vi "Hanging.vi"(9 "Pneumatics In":T2={"CompressorDevRef"={"DevStatus"={"status"=FALSE, "code"=0, "source"=""}, "Pneumatics Control Module"=0}, "High and Low Gear DoubleSolenoidDevRef"={"DevStatus"={"status"=FALSE, "code"=0, "source"=""}, "Pneumatics Control Module"=0, "Forward Solenoid Channel"=enum."Invalid", "Reverse Solenoid Channel"=enum."Invalid"}, "PTO SolenoidDevRef"={"DevStatus"={"status"=FALSE, "code"=0, "source"=""}, "Pneumatics Control Module"=0, "Forward Solenoid Channel"=enum."Invalid", "Reverse Solenoid Channel"=enum."Invalid"}, "Hang Pin SolenoidDevRef"={"DevStatus"={"status"=FALSE, "code"=0, "source"=""}, "Pneumatics Control Module"=0, "Forward Solenoid Channel"=enum."Invalid", "Reverse Solenoid Channel"=enum."Invalid"}}, 11 "Hanging":T13={"Left Erection MotorControlDeviceRef"={"DeviceStatus"={"status"=FALSE, "code"=0, "source"=""}, "Type"=enum."PWM", "PWM"={"PWM Channel"=enum."Invalid", "DeadBand"={"Name"="", "maxPositivePwm"=0, "minPositivePwm"=0, "centerPwm"=0, "maxNegativePwm"=0, "minNegativePwm"=0, "angularRange"=0}}, "CAN"={"Device Number"=0, "Control Mode"=enum."Percent VBus", "Semaphore"=refnum, "Max Vout"=12.0, "TalonSRX Control Mode"=enum."Percent VBus"}, "Invert"=FALSE}, "Right Erection MotorControlDeviceRef"={"DeviceStatus"={"status"=FALSE, "code"=0, "source"=""}, "Type"=enum."PWM", "PWM"={"PWM Channel"=enum."Invalid", "DeadBand"={"Name"="", "maxPositivePwm"=0, "minPositivePwm"=0, "centerPwm"=0, "maxNegativePwm"=0, "minNegativePwm"=0, "angularRange"=0}}, "CAN"={"Device Number"=0, "Control Mode"=enum."Percent VBus", "Semaphore"=refnum, "Max Vout"=12.0, "TalonSRX Control Mode"=enum."Percent VBus"}, "Invert"=FALSE}}) -> (1 "Pneumatics Out":T2={"CompressorDevRef"={"DevStatus"={"status"=FALSE, "code"=0, "source"=""}, "Pneumatics Control Module"=0}, "High and Low Gear DoubleSolenoidDevRef"={"DevStatus"={"status"=FALSE, "code"=0, "source"=""}, "Pneumatics Control Module"=0, "Forward Solenoid Channel"=enum."Invalid", "Reverse Solenoid Channel"=enum."Invalid"}, "PTO SolenoidDevRef"={"DevStatus"={"status"=FALSE, "code"=0, "source"=""}, "Pneumatics Control Module"=0, "Forward Solenoid Channel"=enum."Invalid", "Reverse Solenoid Channel"=enum."Invalid"}, "Hang Pin SolenoidDevRef"={"DevStatus"={"status"=FALSE, "code"=0, "source"=""}, "Pneumatics Control Module"=0, "Forward Solenoid Channel"=enum."Invalid", "Reverse Solenoid Channel"=enum."Invalid"}}, 3 "Hanging":T13={"Left Erection MotorControlDeviceRef"={"DeviceStatus"={"status"=FALSE, "code"=0, "source"=""}, "Type"=enum."PWM", "PWM"={"PWM Channel"=enum."Invalid", "DeadBand"={"Name"="", "maxPositivePwm"=0, "minPositivePwm"=0, "centerPwm"=0, "maxNegativePwm"=0, "minNegativePwm"=0, "angularRange"=0}}, "CAN"={"Device Number"=0, "Control Mode"=enum."Percent VBus", "Semaphore"=refnum, "Max Vout"=12.0, "TalonSRX Control Mode"=enum."Percent VBus"}, "Invert"=FALSE}, "Right Erection MotorControlDeviceRef"={"DeviceStatus"={"status"=FALSE, "code"=0, "source"=""}, "Type"=enum."PWM", "PWM"={"PWM Channel"=enum."Invalid", "DeadBand"={"Name"="", "maxPositivePwm"=0, "minPositivePwm"=0, "centerPwm"=0, "maxNegativePwm"=0, "minNegativePwm"=0, "angularRange"=0}}, "CAN"={"Device Number"=0, "Control Mode"=enum."Percent VBus", "Semaphore"=refnum, "Max Vout"=12.0, "TalonSRX Control Mode"=enum."Percent VBus"}, "Invert"=FALSE}})   [LabVIEW 2015]
uses:
  <vilib>/Rock Robotics/WPI/MotorControl/WPI_MotorControlDeviceRef.ctl
  <vilib>/Rock Robotics/WPI/MotorControl/WPI_MotorControlType.ctl
  <vilib>/Rock Robotics/SystemInterfaces/DIO/FPGA_DIOPWMChannel.ctl
  <vilib>/Rock Robotics/WPI/PWM/WPI_PWMDeadband.ctl
  <vilib>/Rock Robotics/WPI/CAN/Jaguar/SubVIs/WPI_CANJaguar_ControlMode.ctl
  <vilib>/Rock Robotics/WPI/CAN/TalonSRX/WPI_CANTalonSRX_APIControlMode.ctl
  Pnematics.ctl
  <vilib>/Rock Robotics/WPI/Compressor/WPI_CompressorDevRef.ctl
  <vilib>/Rock Robotics/WPI/Solenoid/WPI_SolenoidDevRef.ctl
  <vilib>/Rock Robotics/WPI/Solenoid/WPI_SolenoidChannel.ctl
  <vilib>/Rock Robotics/WPI/Solenoid/WPI_SolenoidValue.ctl
  Robot Values.vi
  <vilib>/Rock Robotics/Network Tables/NT Write String.vi
  <vilib>/Rock Robotics/WPI/Solenoid/WPI_SolenoidSetEnum.vi
  <vilib>/ptbypt/NI_PtbyPt.lvlib
panel:
  out "Right pivot encoder":dbl
  out "Left pivot encoder":dbl
  in  "Pin In":T1=enum."Reverse"
  in  "Pin Out":T1=enum."Forward"
  in  "PTO OUT":T1=enum."Forward"
  in  "PTO IN":T1=enum."Reverse"
  out "encoder offset":dbl
  in  "Setpoint":dbl=100.0
  # "THESE VALUES NEED TO BE UPDATED"
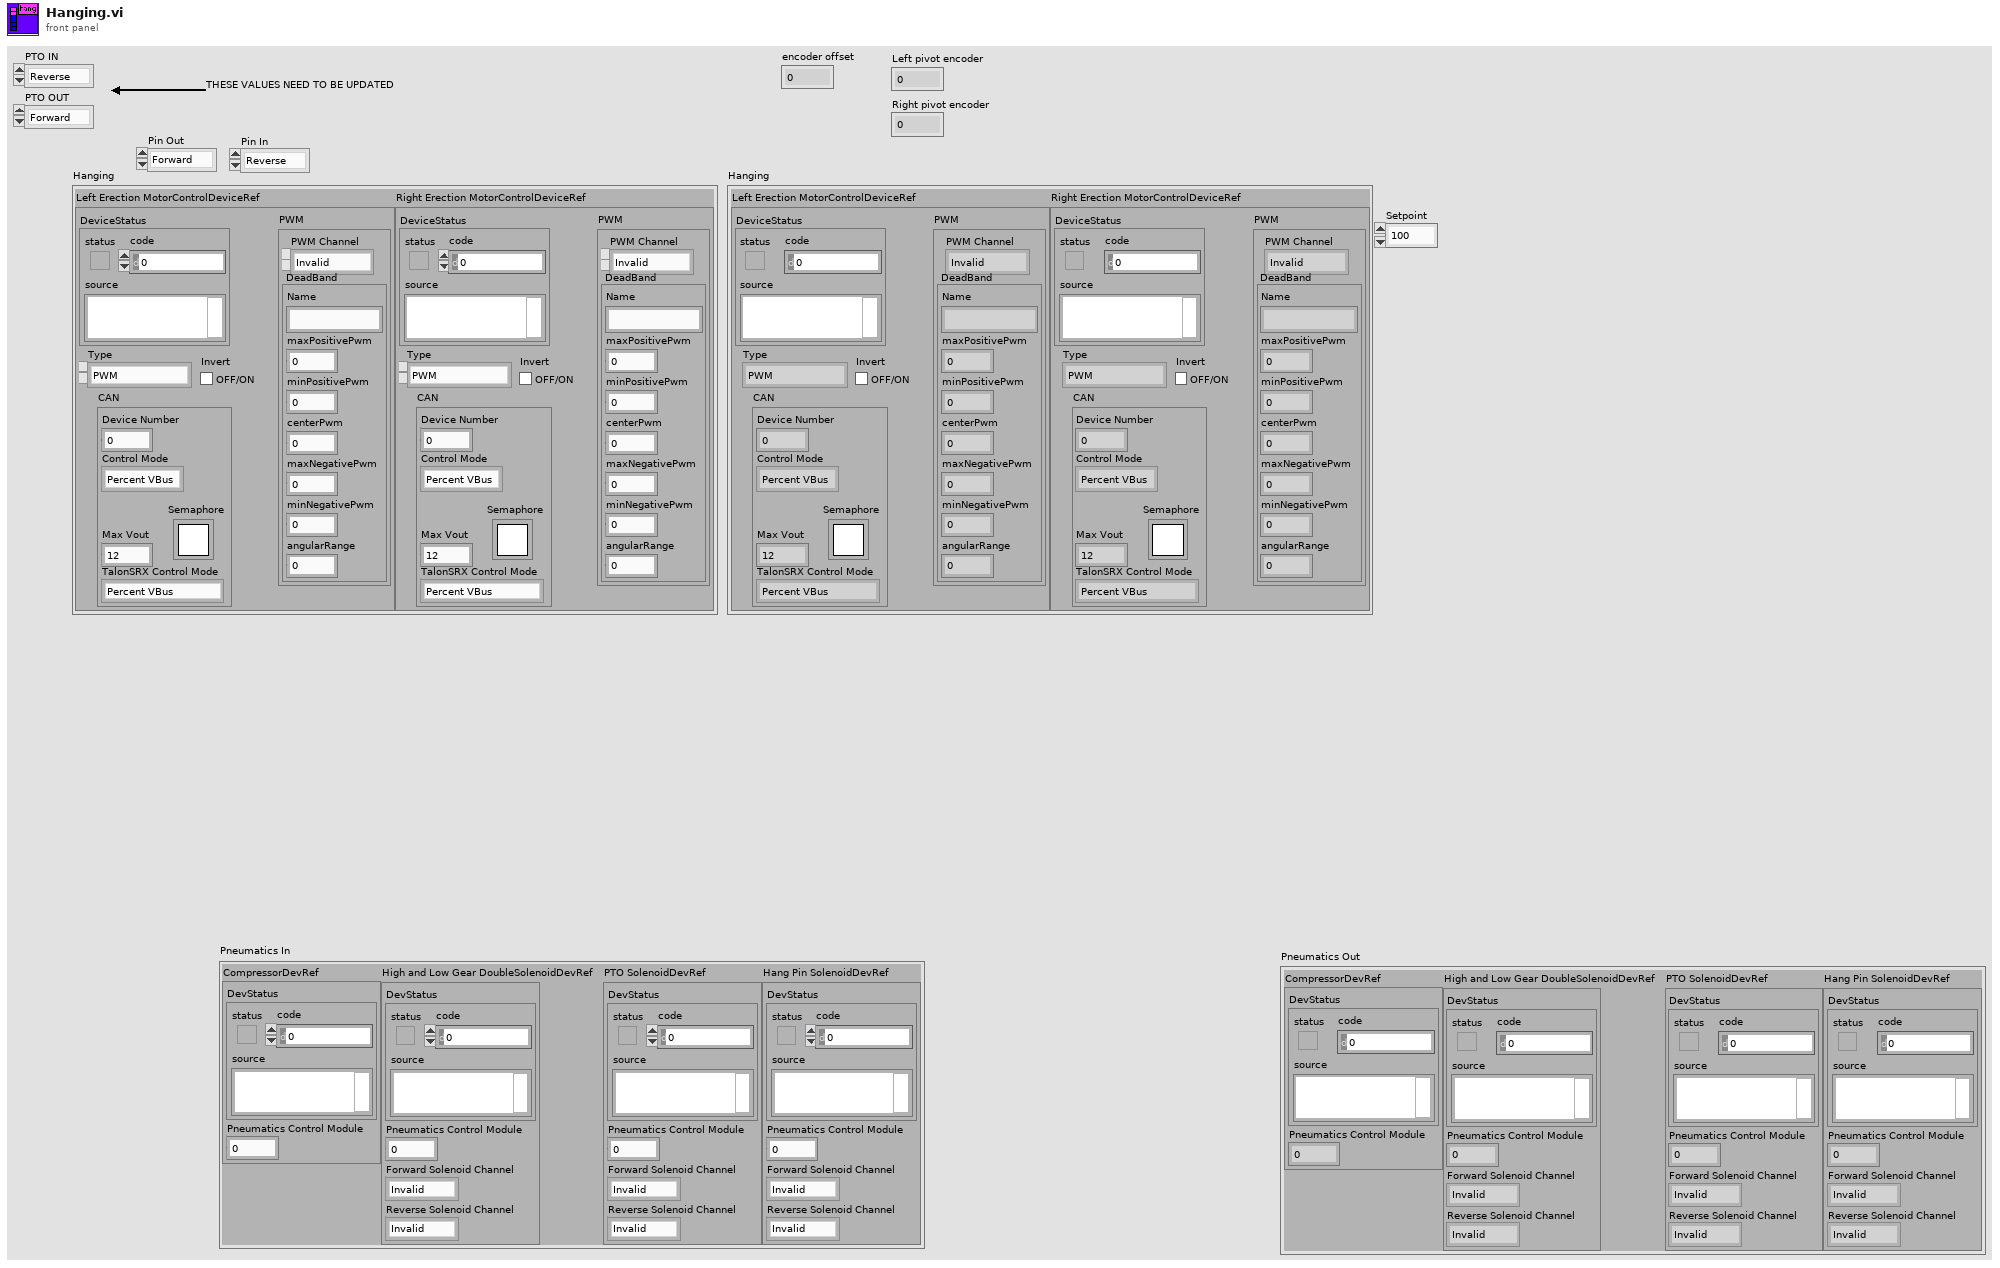
[diagram p1: front panel]
types:
  T1 = typedef "WPI_SolenoidValue.ctl" = enum16{"Off", "On", "Forward", "Reverse"}
  T2 = typedef "Pnematics.ctl" = cluster{"CompressorDevRef":T3, "High and Low Gear DoubleSolenoidDevRef":T4, "PTO SolenoidDevRef":T4, "Hang Pin SolenoidDevRef":T4}
  T3 = typedef "WPI_CompressorDevRef.ctl" = cluster{"DevStatus":errorcluster, "Pneumatics Control Module":u8}
  T4 = typedef "WPI_SolenoidDevRef.ctl" = cluster{"DevStatus":errorcluster, "Pneumatics Control Module":u8, "Forward Solenoid Channel":T5, "Reverse Solenoid Channel":T5}
  T5 = typedef "WPI_SolenoidChannel.ctl" = enum8{"Solenoid 0", "Solenoid 1", "Solenoid 2", "Solenoid 3", "Solenoid 4", "Solenoid 5", "Solenoid 6", "Solenoid 7", "Invalid"}
  T6 = typedef "WPI_MotorControlDeviceRef.ctl" = cluster{"DeviceStatus":errorcluster, "Type":T7, "PWM":cluster{"PWM Channel":T8, "DeadBand":T9}, "CAN":cluster{"Device Number":u8, "Control Mode":T10, "Semaphore":T11, "Max Vout":dbl, "TalonSRX Control Mode":T12}, "Invert":bool}
  T7 = typedef "WPI_MotorControlType.ctl" = enum16{"PWM", "CAN", "CANTalonSRX"}
  T8 = typedef "FPGA_DIOPWMChannel.ctl" = enum8{"PWM 0", "PWM 1", "PWM 2", "PWM 3", "PWM 4", "PWM 5", "PWM 6", "PWM 7", "PWM 8", "PWM 9", "PWM MXP 0", "PWM MXP 1", "PWM MXP 2", "PWM MXP 3", "PWM MXP 4", "PWM MXP 5", "PWM MXP 6", "PWM MXP 7", "PWM MXP 8", "PWM MXP 9", "Invalid"}
  T9 = typedef "WPI_PWMDeadband.ctl" = cluster{"Name":string, "maxPositivePwm":i32, "minPositivePwm":i32, "centerPwm":i32, "maxNegativePwm":i32, "minNegativePwm":i32, "angularRange":u16}
  T10 = typedef "WPI_CANJaguar_ControlMode.ctl" = enum8{"Percent VBus", "Current", "Speed", "Position", "Voltage"}
  T11 = typedef "Semaphore RefNum" = refnum<k1>
  T12 = typedef "WPI_CANTalonSRX_APIControlMode.ctl" = enum8{"Percent VBus", "Speed", "Position", "Slave", "Unchanged / Invalid", "Voltage Compensation", "Current", "Motion Profile"}
  T13 = cluster{"Left Erection MotorControlDeviceRef":T6, "Right Erection MotorControlDeviceRef":T6}
  T14 = typedef "Robot Values.ctl" = cluster{"Drive Motors":cluster{"Left Motor Value":dbl, "Right Motor Value":dbl, "Left Motor Encoder":dbl, "Right Motor Encoder":dbl, "High/Low Gear":bool}, "Sensors":cluster{"Gyro Angle":dbl, "Photoeye":bool, "Ultrasonic Range":dbl, "Shooter Speed Encoder":dbl, "Accelerometer Value":dbl, "Flashlight":bool, "Target Distance":dbl, "Target X Value":dbl, "Reset Gyro?":bool}, "Arms":cluster{"Desired Arm Position":dbl, "Left Arm Encoder":dbl, "Right Arm Encoder":dbl, "Left Arm Lower Limit":bool, "Right Arm Lower Limit":bool, "Initialize Arm Position?":bool}, "Acquisition and Scoring":cluster{"Acquiring?":bool, "Current Speed":dbl, "Setpoint Speed":dbl, "Prep Wheels":bool, "Shoot":bool, "Low Eject":bool, "Reverse Shooter Wheel":bool}, "Hanging":cluster{"Pivot Arms":dbl, "PTO":bool, "Left Pivot Encoder":dbl, "Right Pivot Encoder":dbl, "Hanging Pin":bool}}
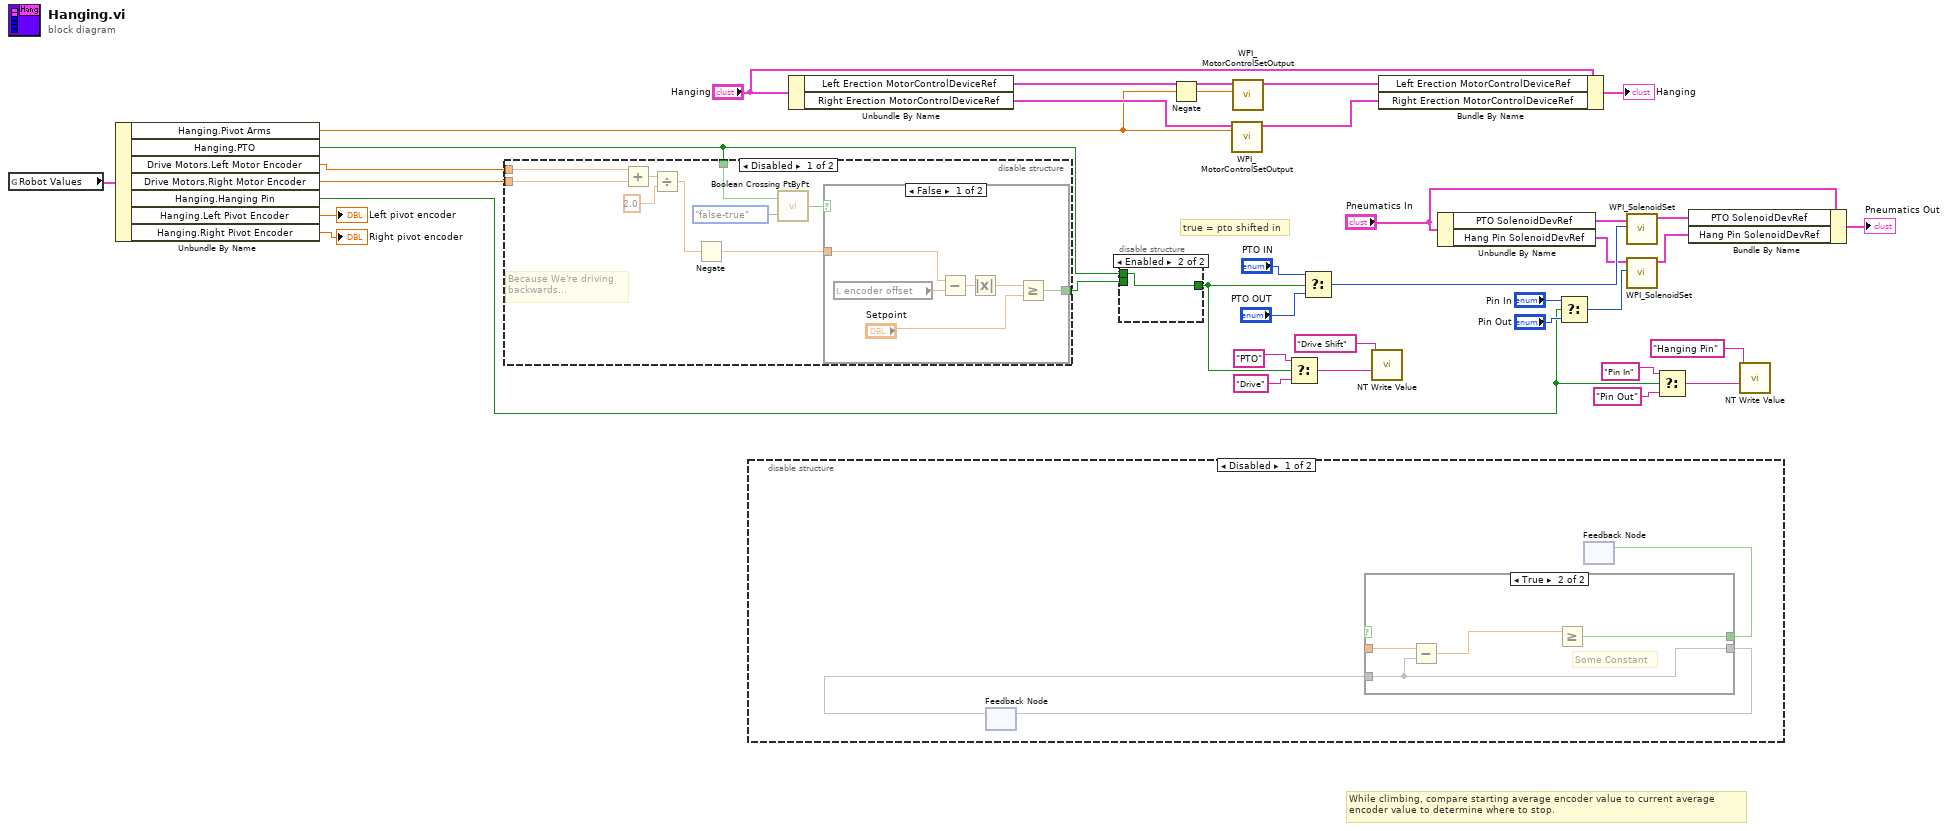
[diagram p0: block diagram]
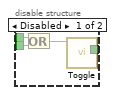
[diagram p2: hidden frame]
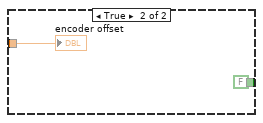
[diagram p3: hidden frame]
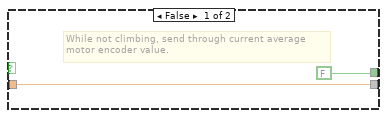
[diagram p5: hidden frame]
diagram:
  # "true = pto shifted in"
  # "While climbing, compare starting average encoder value to current average\nencoder value to determine where to stop."
  n1 = global read "Robot Values.vi" "Robot Values"() -> (w31:T14)
  n2 = Unbundle By Name(w31) -> ("Hanging.Pivot Arms"=w30:dbl, "Hanging.PTO"=w17:bool, "Drive Motors.Left Motor Encoder"=w22:dbl, "Drive Motors.Right Motor Encoder"=w21:dbl, "Hanging.Hanging Pin"=w1:bool, "Hanging.Left Pivot Encoder"=→"Left pivot encoder":dbl, "Hanging.Right Pivot Encoder"=→"Right pivot encoder":dbl)
  n3 = disable-structure shown="Disabled" {
    disable-tunnel: w22 -> [w47 _]
    disable-tunnel: w21 -> [w46 _]
    disable-tunnel: w17 -> [w43 _]
    disable-tunnel: [w40 _] -> w16
    frame Disabled {
      # "Because We're driving \nbackwards..."
      n4 = Add(x=w47, y=w46) -> (x+y=w45:dbl)
      n5 = Divide(x=w45, y=2.0) -> (x/y=w39:dbl)
      n6 = Negate(x=w39) -> (-x=w38:dbl)
      n7 = call <vilib>:"Boolean Crossing PtByPt.vi"("direction"=enum16{"either", "false-true", "true-false"}."false-true", "input"=w43) -> ("crossing"=w41:bool)  [unwired: 1 in]
      n8 = case shown="False" w41 {
        tunnel: w38 -> [w52 w55]
        tunnel: [w50 FALSE] -> w40
        frame False {
          n9 = local read "encoder offset"() -> (w53:dbl)
          n10 = Subtract(x=w52, y=w53) -> (x-y=w51:dbl)
          n11 = Absolute Value(x=w51) -> (abs(x)=w49:dbl)
          n12 = Greater Or Equal?(x=w49, y="Setpoint") -> (x >= y?=w50:bool)
        }
        frame True {
          "encoder offset" <- w55
        }
      }
    }
    frame Enabled {
    }
  }
  n13 = disable-structure shown="Disabled" {
    frame Disabled {
      n14 = feedback #1() -> (w57)  [unwired: 1 in]
      n15 = case shown="True" {
        selector: _ -> [_ _]
        tunnel: _ -> [w60 w65]
        tunnel: [w60 w64] -> w58
        tunnel: w57 -> [_ w64]
        tunnel: [FALSE w61] -> w56
        frame False {
          # "While not climbing, send through current average\nmotor encoder value."
        }
        frame True {
          # "Some Constant"
          n16 = Subtract(x=w65, y=w64) -> (x-y=w63:dbl)
          n17 = Greater Or Equal?(x=w63) -> (y=w62:dbl, x >= y?=w61:bool)
        }
      }
      n18 = feedback-in #1(w58) -> ()
      n19 = feedback #2() -> ()  [unwired: 2 in]
      n20 = feedback-in #2(w56) -> ()
    }
    frame Enabled {
    }
  }
  n21 = Unbundle By Name("Hanging") -> ("Left Erection MotorControlDeviceRef"=w35:T6, "Right Erection MotorControlDeviceRef"=w33:T6)
  n22 = disable-structure shown="Enabled" {
    disable-tunnel: [w68 w70] -> w20
    disable-tunnel: w17 -> [w67 w70]
    disable-tunnel: w16 -> [w66 _]
    frame Disabled {
      n23 = Or(x=w67, y=w66) -> (x .or. y?=w69:bool)
      n24 = call "Toggle.vi"("Input"=w69) -> ("output"=w68:bool)  [unwired: 10 in]
    }
    frame Enabled {
    }
  }
  n25 = Negate(x=w30) -> (-x=w11:dbl)
  n26 = call <vilib>:"WPI_MotorControlSetOutput.vi"("Output"=w30, "MotorControlDevRef"=w33) -> ("MotorControlDevRef"=w32:T6)  [unwired: 7 in, 2 out]
  n27 = call <vilib>:"WPI_MotorControlSetOutput.vi"("Output"=w11, "MotorControlDevRef"=w35) -> ("MotorControlDevRef"=w34:T6)  [unwired: 7 in, 2 out]
  n28 = Select(t="PTO", s=w20, f="Drive") -> (s? t:f=w24:string)
  n29 = Select(t="PTO IN", s=w20, f="PTO OUT") -> (s? t:f=w26:T1)
  n30 = call-poly <vilib>:"NT Write Value.vi"("String"=w24, "Name"="Drive Shift") -> ()  [unwired: 9 in, 1 out]
  n31 = Bundle By Name(cluster="Hanging", "Left Erection MotorControlDeviceRef"=w34, "Right Erection MotorControlDeviceRef"=w32) -> (→"Hanging":T13)
  n32 = Unbundle By Name("Pneumatics In") -> ("PTO SolenoidDevRef"=w27:T4, "Hang Pin SolenoidDevRef"=w15:T4)
  n33 = Select(t="Pin In", s=w1, f="Pin Out") -> (s? t:f=w12:T1)
  n34 = call-poly <vilib>:"WPI_SolenoidSet.vi"("Value"=w26, "SolenoidDevRef"=w27) -> ("SolenoidDevRef"=w25:T4)  [unwired: 8 in, 1 out]
  n35 = call-poly <vilib>:"WPI_SolenoidSet.vi"("Value"=w12, "SolenoidDevRef"=w15) -> ("SolenoidDevRef"=w6:T4)  [unwired: 8 in, 1 out]
  n36 = Select(t="Pin In", s=w1, f="Pin Out") -> (s? t:f=w5:string)
  n37 = Bundle By Name(cluster="Pneumatics In", "PTO SolenoidDevRef"=w25, "Hang Pin SolenoidDevRef"=w6) -> (→"Pneumatics Out":T2)
  n38 = call-poly <vilib>:"NT Write Value.vi"("String"=w5, "Name"="Hanging Pin") -> ()  [unwired: 9 in, 1 out]
